vi "FromRepo.vi"(8 "error in":errorcluster, 9 "from repo cluster":T2, 10 "repository in":refnum<class "NISE_CEF_Repository.lvclass">, 11 "channel in":refnum<class "Channel.lvclass">) -> (0 "error out":errorcluster, 2 "repository out":refnum<class "NISE_CEF_Repository.lvclass">, 3 "node":T1)   [LabVIEW 2013, in "Channel.lvclass"]
uses:
  Channel.lvclass
  Configuration Framework/Repository/NISE_CEF_Repository.lvclass
  Configuration Framework/Node/FromRepoCluster.ctl
  Configuration Framework/Node/NodeRef.ctl
  Configuration Framework/Node/NISE_CEF_Node.lvclass
  cRIO Repo/cRIORepo.lvclass
  cRIO Repo/cRIORepo.lvclass/cRIORepo.ctl
  Channel.lvclass/Channel.ctl
  cRIO Repo/Read Channels.vi
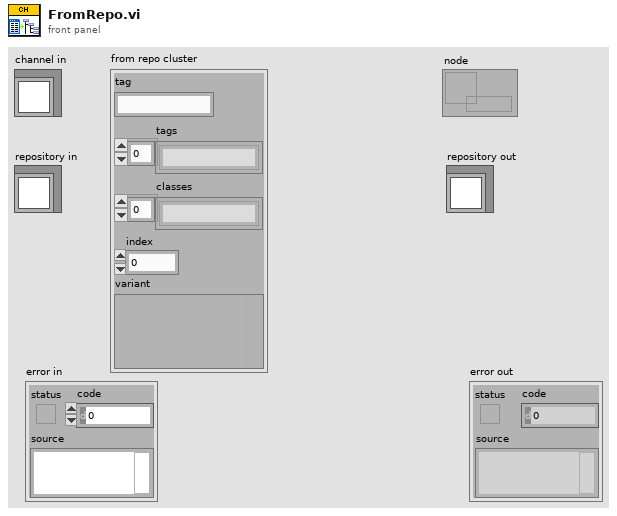
[diagram p1: front panel]
types:
  T1 = typedef "NISE_CEF_Node.lvclass/NodeRef.ctl" = refnum<data-value>
  T2 = typedef "NISE_CEF_Node.lvclass/FromRepoCluster.ctl" = cluster{"tag":string, "tags":string[], "classes":string[], "index":i32, "variant":variant}
  T3 = typedef "Channel.ctl" = cluster{"channel group":string, "channel name":string, "IO ":string, "sensor ID":string, "description":string, "system":string, "channel type":string}
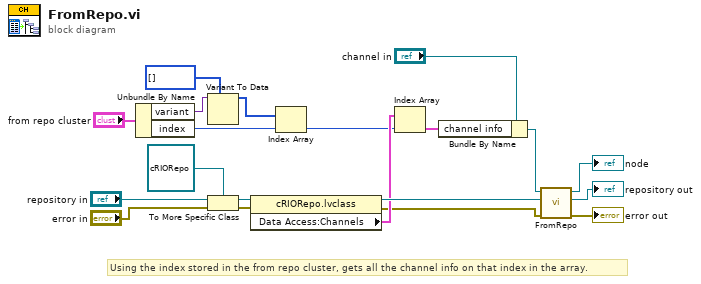
[diagram p0: block diagram]
diagram:
  # "Using the index stored in the from repo cluster, gets all the channel info on that index in the array."
  n1 = Unbundle By Name("from repo cluster") -> ("variant"=w14:variant, "index"=w11:i32)
  n2 = Variant To Data(type=i32[] [], Variant=w14) -> (data=w12:i32[])  [unwired: 1 in, 1 out]
  n3 = To More Specific Class(target class=refnum<class "cRIORepo.lvclass"> refnum ("cRIO repo.lvclass"), reference="repository in", error in="error in") -> (specific class reference=w8:refnum<class "cRIORepo.lvclass">, error out=w1:errorcluster)
  n4 = property class="cRIORepo.lvclass"(reference=w8, error in=w1) -> (reference out=w7:refnum<class "cRIORepo.lvclass">, error out=w3:errorcluster, "Data Access:Channels"=w6:T3[])
  n5 = Index Array(array=w12, index=w11) -> (element=w5:i32)
  n6 = Index Array(array=w6, index=w5) -> (element=w4:T3)
  n7 = Bundle By Name(cluster="channel in", "channel info"=w4) -> (w16:refnum<class "Channel.lvclass">)
  n8 = call-parent "FromRepo.vi"("error in"=w3, "repository in"=w7, "node in"=w16) -> ("error out"=→"error out":errorcluster, "repository out"=→"repository out":refnum<class "NISE_CEF_Repository.lvclass">, "node"=→"node":T1)  [unwired: 6 in]
